vi "RP Read RX FIFO Fast TCP.vi"(6 "Samples per read":i32=1024, 7 "bytes per sample":i32=12, 8 "Error In":errorcluster, 11 "connection ID":refnum<k5>) -> (0 "Error Out":errorcluster, 2 "FIFO out":i32[](array[numeric]), 3 "connection ID out":refnum<k5>)   [LabVIEW 2024]
uses:
  RP Command.ctl
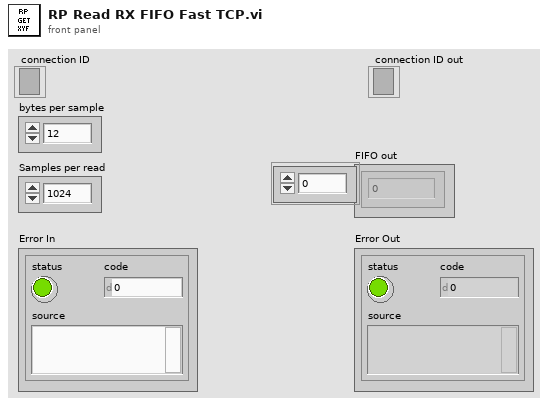
[diagram p1: front panel]
types:
  T1 = typedef "RP Command.ctl" = enum16{"Reset", "Read IDN", "Stop server", "Get status", "Get temperature", "Connect client", "Arm", "Software trigger", "Get whole buffer", "Get chunk", "System call", "Get config", "Set config", "Recieve data", "Recieve Calibartion", "Transmit data"}
  T2 = enum16{"big-endian, network order", "native, host order", "little-endian"}
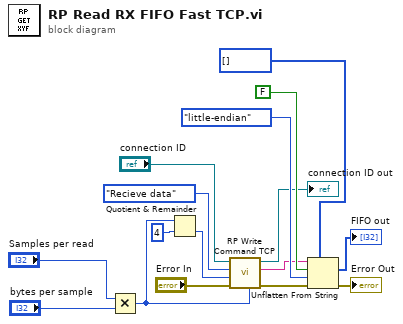
[diagram p0: block diagram]
diagram:
  n1 = Multiply(x="Samples per read", y="bytes per sample") -> (x*y=w4:i32)
  n2 = Quotient & Remainder(x=w4, y=4) -> (floor(x/y)=w5:i32)  [unwired: 1 out]
  n3 = call "RP Write Command TCP.vi"("bytes to read"=w4, "Error In"="Error In", "Command payload"=w5, "Command number"=RP_Command."Recieve data", "connection ID"="connection ID") -> ("Error Out"=w1:errorcluster, "data out"=w3:string, "connection ID out"=→"connection ID out":refnum<k5>)  [unwired: 3 in, 1 out]
  n4 = Unflatten From String(type=i32[] [], binary string=w3, data includes array or string size? (T)=FALSE, byte order (0:big-endian, network order)=T2."little-endian", error in (no error)=w1) -> (value=→"FIFO out":i32[], error out=→"Error Out":errorcluster)  [unwired: 1 out]
